vi "URAPI_InitTimer_num.vi"(0 "Variable In":string="timer", 3 "URAPI Script":T1={"Script"="", "Whiles"=[], "Ifs"=[], "Supress Err"=TRUE, "Errors"=""}, 4 "Timer":u8) -> (2 "Variable out":string="timer", 5 "URAPI Script out":T1={"Script"="", "Whiles"=[], "Ifs"=[], "Supress Err"=TRUE, "Errors"=""})   [LabVIEW 2012]
doc: "Initializes the timer associated with the unique \"Timer\" value."
uses:
  <userlib>/BotSpeak/VIs/Direct/URAPI_Control.ctl
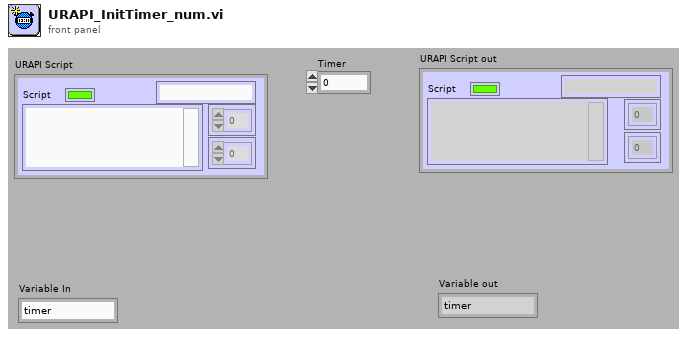
[diagram p1: front panel]
types:
  T1 = typedef "URAPI_Control.ctl" = cluster{"Script":string, "Whiles":u8[], "Ifs":u8[], "Supress Err":bool, "Errors":string}
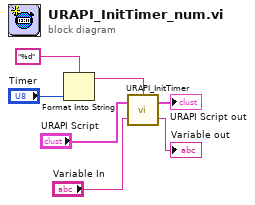
[diagram p0: block diagram]
diagram:
  n1 = Format Into String(format string="%d" ("string"), "Timer") -> (resulting string=w1:string)  [unwired: 2 in, 1 out]
  n2 = call <userlib>:"URAPI_InitTimer.vi"("Variable In"="Variable In", "URAPI Script"="URAPI Script", "Timer"=w1) -> ("Variable out"=→"Variable out":string, "URAPI Script out"=→"URAPI Script out":T1)  [unwired: 1 in]
